vi "Batch Do.vi"(7 "Priority":u16, 8 "error in (no error)":errorcluster, 9 "Message Array in":refnum<class "Message.lvclass">[](array[class]), 10 "Sequencer in":refnum<class "Sequencer.lvclass">, 11 "Multi Instrument Batch Msg":refnum<class "Multi Instrument Batch Msg.lvclass">) -> (0 "error out":errorcluster, 2 "Sequencer out":refnum<class "Sequencer.lvclass">)   [LabVIEW 2020, in "Instrument Handler.lvlib" / "Multi Instrument Batch Msg.lvclass"]
doc: "Act on the Batch message array.\n\nThe default implementation enqueues the message array in front on the Sequencer Core."
uses:
  Multi Instrument Batch Msg.lvclass
  PPL/HDH.Actor Framework.Core.Actor.lvlibp/1abvi3w/vi.lib/ActorFramework/Message/Message.lvclass
  PPL/HDH.Actor Framework.Core.Sequencer.lvlibp/Sequencer/Sequencer.lvclass
  C:/Current projects/WS/PPL/HDH.Actor Framework.Core.Actor.lvlibp/1abvi3w/vi.lib/ActorFramework/Actor/Actor.lvclass
  Multi Instrument Batch Msg.lvclass/Multi Instrument Batch Msg.ctl
  Custom Multi Instrument Msg/Custom Multi Instrument Msg.lvclass/Custom Multi Instrument Msg.ctl
  Messages/Instrument Msg/Instrument Msg.lvclass/Instrument Msg.ctl
  Custom Multi Instrument Msg/Custom Multi Instrument Msg.lvclass
  C:/Current projects/WS/Framework/Framework/Actors/Instrument Handler/Messages/Instrument Msg/Instrument Msg.lvclass
  Messages/Instrument Msg/Instrument Msg.lvclass
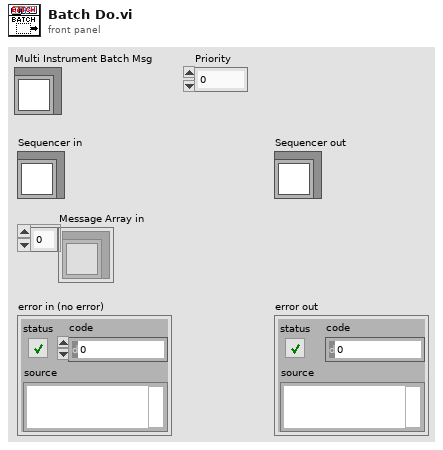
[diagram p1: front panel]
types:
  T1 = typedef "HDH.Actor Framework.Core.Publisher.lvlibp/Ctl_SendFunction.ctl" = enum16{"Send and Forget", "Request Reply", "Await Reply"}
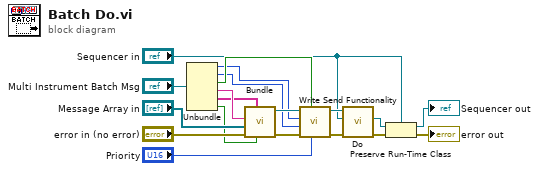
[diagram p0: block diagram]
diagram:
  n1 = Unbundle("Multi Instrument Batch Msg") -> (w16:T1, w15:i32, w17:bool, w12:string, w11:string[], w1:bool)
  n2 = call "Bundle.vi"("Combined Publish?"=w1, "Data Alias Array"=w11, "error in (no error)"="error in (no error)", "Message Array in"="Message Array in", "Msg Alias"=w12) -> ("error out"=w14:errorcluster, "Reorder Driver Aliases Msg out"=w18:refnum<class "Custom Multi Instrument Msg.lvclass">)  [unwired: 5 in]
  n3 = call "Write Send Functionality.vi"("Message Priority(Normal)"="Priority", "Publish Data?(T)"=w17, "error in (no error)"=w14, "Timeout if Waiting(-1ms)"=w15, "Send Function(Await Reply)"=w16, "Instrument Msg in"=w18) -> ("error out"=w5:errorcluster, "Instrument Msg out"=w9:refnum<class "Custom Multi Instrument Msg.lvclass">)  [unwired: 4 in]
  n4 = call-dynamic "Do.vi"("error in (no error)"=w5, "Actor in"="Sequencer in", "Instrument Msg"=w9) -> ("error out"=w7:errorcluster, "Actor out"=w8:refnum<class "Actor.lvclass">)  [unwired: 7 in]
  n5 = Preserve Run-Time Class(object in=w8, error in=w7, 2:"Sequencer in") -> (object out=→"Sequencer out":refnum<class "Sequencer.lvclass">, error out=→"error out":errorcluster)
